vi "AlazarBoardsInSystemBySystemID.vi"(0 "System ID":u32, 1 "error in (no error)":errorcluster) -> (2 "Board Count":u32, 3 "Return Code":u32, 4 "error out":errorcluster)   [LabVIEW 2009]
doc: "Return the number of digitizer boards in a board system specified its system ID.s"
uses:
  ATSApi.dll
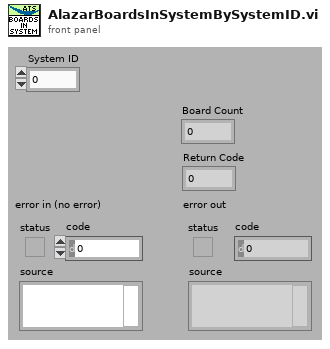
[diagram p1: front panel]
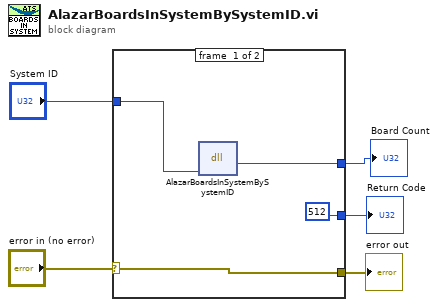
[diagram p0: block diagram]
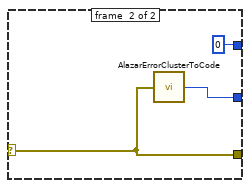
[diagram p2: hidden frame]
diagram:
  n1 = case shown="No Error" "error in (no error)" {
    selector: "error in (no error)" -> [w8 w12]
    tunnel: [w8 w12] -> w4
    tunnel: [u32 512 w11] -> w3
    tunnel: "System ID" -> [w9 _]
    tunnel: [w6 u32 0] -> w1
    frame #0 {
      n2 = dll-call lib="ATSApi.dll" fn="AlazarBoardsInSystemBySystemID"("systemIDs"=w9) -> (w6:u32)  [unwired: 4 in, 2 out]
    }
    frame #1 {
      n3 = call "AlazarErrorClusterToCode.vi"("error in (no error)"=w12) -> ("Error Code"=w11:u32)
    }
  }
  "error out" <- w4
  "Return Code" <- w3
  "Board Count" <- w1
